vi "Resample N Waveforms (single shot).vi"(0 "waveforms in":waveform(dbl)[](array[waveform]), 1 "open interval? (F)":bool, 5 "dt":dbl=1.0 format="%.2p", 7 "t0":timestamp=timestamp(-9223372036854775808 s since 1904-01-01) format="%<%.4X>T", 9 "interpolation mode":u16(ring)=1 items=["coerce", "linear", "spline", "FIR filter"], 11 "error in (no error)":errorcluster, 12 "FIR filter specifications":T1={"alias rejection (dB)"=120.0, "normalized bandwidth"=0.4536} {"normalized bandwidth" format="%.4f"; "alias rejection (dB)" format="%.2f"}) -> (4 "resampled waveforms out":waveform(dbl)[](array[waveform]), 10 "used t0's":timestamp[](array[timestamp]) format="%<%.4X>T", 14 "t0 adjusted warnings":bool[](array[boolean]), 15 "error out":errorcluster)   [LabVIEW 2020, in "NI_MAPro.lvlib"]
doc: "Resamples input waveforms or data according to the user-defined <B>t0</B> and <B>dt</B> values.\n\nWire data to the waveform or data input to determine the polymorphic instance to use or manually select the instance."
uses:
  NI_MAPro.lvlib
panel:
  # "open"
  # "closed"
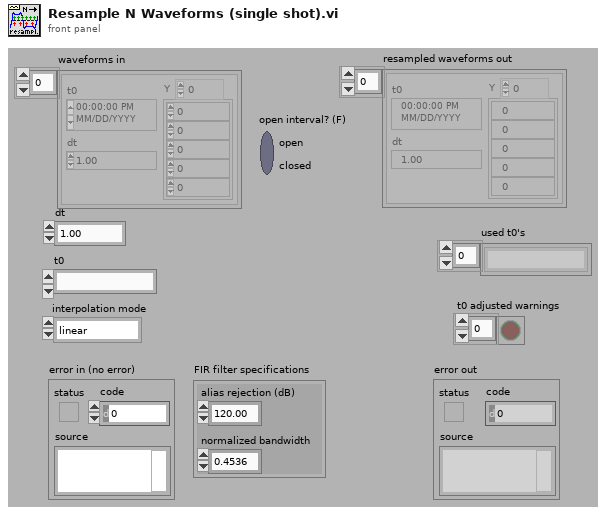
[diagram p1: front panel]
types:
  T1 = cluster{"alias rejection (dB)":dbl, "normalized bandwidth":dbl}
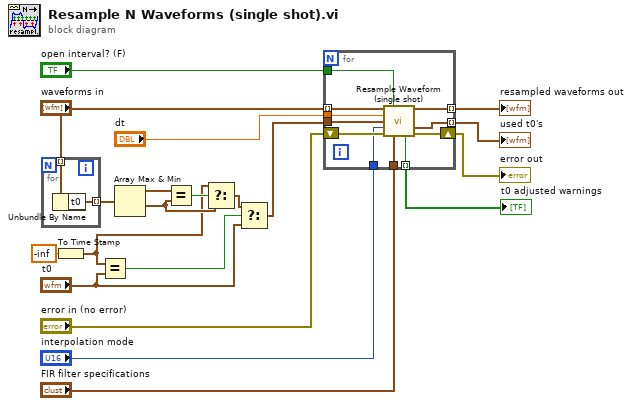
[diagram p0: block diagram]
diagram:
  n1 = for {
    tunnel: "waveforms in" -> [w22] mode=indexing
    tunnel: [w21] -> w10 mode=indexing
    n2 = Unbundle By Name(w22) -> ("t0"=w21:timestamp)
  }
  n3 = To Time Stamp(1:-inf ("x")) -> (0:w1:timestamp)
  n4 = Equal?(x=w1, y="t0") -> (x = y?=w6:bool)
  n5 = Array Max & Min(array=w10) -> (max value=w4:timestamp, min value=w3:timestamp)  [unwired: 2 out]
  n6 = Equal?(x=w4, y=w3) -> (x = y?=w5:bool)
  n7 = Select(t=w1, s=w5, f=w3) -> (s? t:f=w2:timestamp)
  n8 = Select(t=w2, s=w6, f="t0") -> (s? t:f=w9:timestamp)
  n9 = for {
    tunnel: "waveforms in" -> [w33] mode=indexing
    shift-right: [w31] -> w19
    shift-left: "error in (no error)" -> [w32]
    tunnel: [w30] -> w18 mode=indexing
    tunnel: [w29] -> w17 mode=indexing
    tunnel: [w28] -> w16 mode=indexing
    tunnel: "dt" -> [w27]
    tunnel: w9 -> [w26]
    tunnel: "interpolation mode" -> [w24]
    tunnel: "open interval? (F)" -> [w25]
    tunnel: "FIR filter specifications" -> [w23]
    n10 = call "Resample Waveform (single shot).vi"("waveform in"=w33, "open interval? (F)"=w25, "dt"=w27, "t0"=w26, "interpolation mode"=w24, "error in (no error)"=w32, "FIR filter specifications"=w23) -> ("resampled waveform out"=w29:waveform(dbl), "used t0"=w30:timestamp, "t0 adjusted warning"=w28:bool, "error out"=w31:errorcluster)  [unwired: 5 in]
  }
  "error out" <- w19
  "resampled waveforms out" <- w17
  "used t0's" <- w18
  "t0 adjusted warnings" <- w16
